vi "Build Response Error.vi"(8 "error in (no error)":errorcluster, 9 "message":string, 10 "code":i32, 11 "message id in":i32) -> (0 "error out":errorcluster, 3 "MCP message out":string)   [LabVIEW 2020, in "MCP Server.lvlib"]
doc: "This VI build a JSON container with a field \"jsonrpc\" set to \"2.0\", id set to the number id, and \"error\" set to code + message."
uses:
  MCP Server.lvlib
  aaa441bb-6e8c-4ec0-8711-827d95f5656f.vi
  e71c233f-4ea6-4aba-9a41-f999e1cb3491.vi
  8ee560a3-2e04-4350-9390-df7ad8ca5a93.vi
  8a0140cc-e067-4e92-8974-54f7e9800590.vi
  <vilib>/JDP Science/JSONtext/Variant to JSON Text.vi
  <vilib>/JDP Science/JSONtext/support/Format JSON Object.vi
  <vilib>/JDP Science/JSONtext/LVClass Serializer/JSONtext LVClass Serializer.lvclass
  <vilib>/JDP Science/JSONtext/JSONtext.lvlib
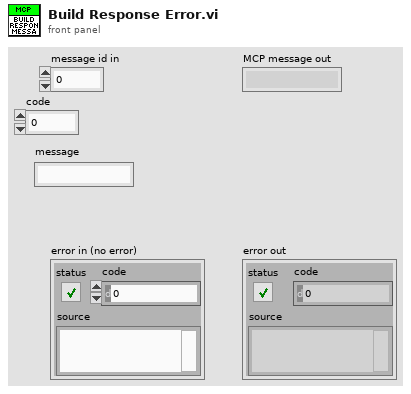
[diagram p1: front panel]
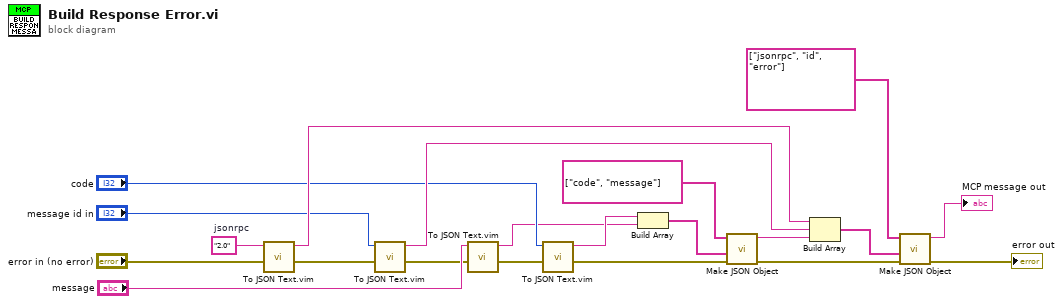
[diagram p0: block diagram]
diagram:
  w15 = "2.0"  # jsonrpc
  n1 = call "To JSON Text.vim"("error in (no error)"="error in (no error)", "Anything"=w15) -> ("error out"=w12:errorcluster, "<JSON>"=w16:string)  [unwired: 8 in]
  n2 = call "To JSON Text.vim"("error in (no error)"=w12, "Anything"="message id in") -> ("error out"=w3:errorcluster, "<JSON>"=w14:string)  [unwired: 8 in]
  n3 = call "To JSON Text.vim"("error in (no error)"=w3, "Anything"="message") -> ("error out"=w2:errorcluster, "<JSON>"=w5:string)  [unwired: 8 in]
  n4 = call "To JSON Text.vim"("error in (no error)"=w2, "Anything"="code") -> ("error out"=w1:errorcluster, "<JSON>"=w9:string)  [unwired: 8 in]
  n5 = Build Array(w9, w5) -> (w8:string[])
  n6 = call <vilib>:"Make JSON Object.vi"("error in (no error)"=w1, "JSON Items"=w8, "Item Names"=string[] ["code", "message"]) -> ("error out"=w11:errorcluster, "<JSON>"=w6:string)  [unwired: 7 in]
  n7 = Build Array(w16, w14, w6) -> (w17:string[])
  n8 = call <vilib>:"Make JSON Object.vi"("error in (no error)"=w11, "JSON Items"=w17, "Item Names"=string[] ["jsonrpc", "id", "error"]) -> ("error out"=→"error out":errorcluster, "<JSON>"=→"MCP message out":string)  [unwired: 7 in]
